vi "Read Location.vi"(8 "error in (no error)":errorcluster, 11 "Food in":refnum<class "Food.lvclass">) -> (0 "error out":errorcluster, 2 "Location":cluster{"x":u32, "y":u32}, 3 "Food out":refnum<class "Food.lvclass">)   [LabVIEW 2020, in "Food.lvclass"]
uses:
  Food.lvclass
  Food.lvclass/Food.ctl
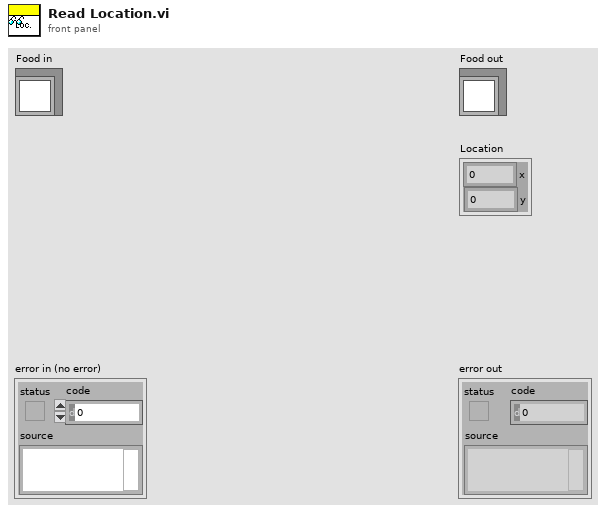
[diagram p1: front panel]
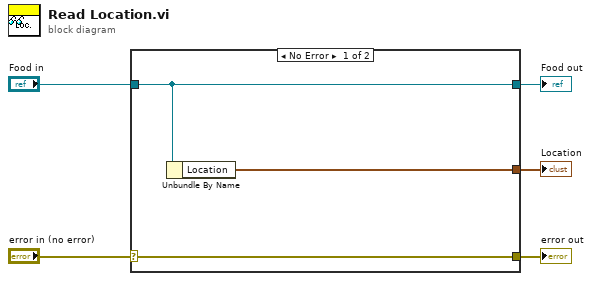
[diagram p0: block diagram]
diagram:
  n1 = case shown="No Error" "error in (no error)" {
    selector: "error in (no error)" -> [w8 w9]
    tunnel: [w8 w9] -> w4
    tunnel: [w7 w10] -> w2
    tunnel: "Food in" -> [w7 w10]
    tunnel: [w6 _] -> w1
    frame No Error {
      n2 = Unbundle By Name(w7) -> ("Location"=w6:cluster{"x":u32, "y":u32})
    }
    frame Error {
    }
  }
  "error out" <- w4
  "Food out" <- w2
  "Location" <- w1
